vi "Get Codec.vi"(8 "error in (no error)":errorcluster, 10 "Codec In":string, 11 "Absolute Path":path) -> (0 "error out":errorcluster, 3 "Codec Out":string)   [LabVIEW 2020, in "G-Audio.lvlib"]
doc: "Determines supported audio codec name based on file extension or wired in codec string."
uses:
  G-Audio.lvlib
  <vilib>/Utility/error.llb/Error Cluster From Error Code.vi
  <vilib>/ErrorRing/Error Ring.xnode
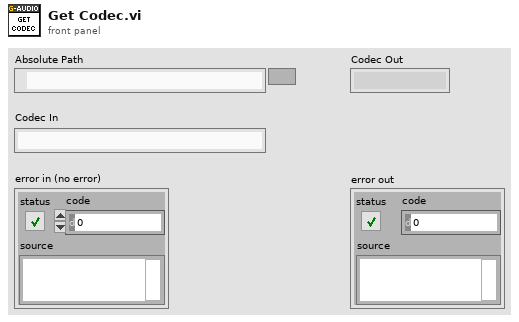
[diagram p1: front panel]
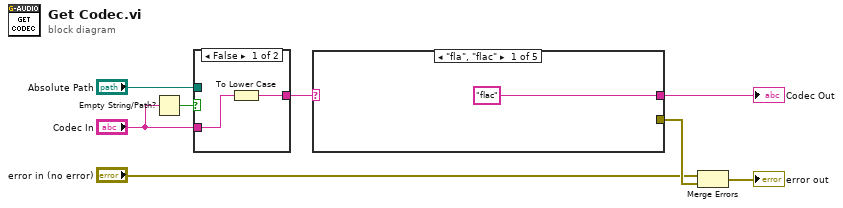
[diagram p0: block diagram]
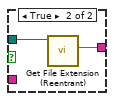
[diagram p2: hidden frame]
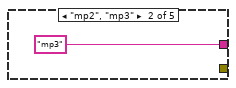
[diagram p3: hidden frame]
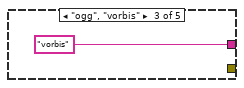
[diagram p4: hidden frame]
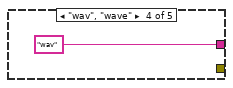
[diagram p5: hidden frame]
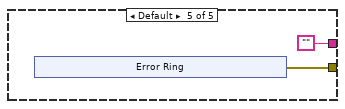
[diagram p6: hidden frame]
diagram:
  n1 = Empty String/Path?(string/path="Codec In") -> (empty?=w8:bool)
  n2 = case shown="False" w8 {
    tunnel: "Absolute Path" -> [_ w12]
    tunnel: [w9 w11] -> w6
    tunnel: "Codec In" -> [w10 _]
    frame False {
      n3 = To Lower Case(string=w10) -> (all lower case string=w9:string)
    }
    frame True {
      n4 = call "Get File Extension (Reentrant).vi"("file"=w12) -> ("lowercase file extension"=w11:string)  [unwired: 6 in, 4 out]
    }
  }
  n5 = case shown="\"fla\", \"flac\"" w6 {
    tunnel: ["flac" ("lowercase file extension") "mp3" ("lowercase file extension") "vorbis" ("lowercase file extension") "wav" ("lowercase file extension") "" ("lowercase file extension")] -> w4
    tunnel: [_ _ _ _ w17] -> w3
    frame "fla", "flac" {
    }
    frame "mp2", "mp3" {
    }
    frame "ogg", "vorbis" {
    }
    frame "wav", "wave" {
    }
    frame Default {
      n6 = xnode ("Error Ring")() -> ("error out"=w17:errorcluster)
    }
  }
  "Codec Out" <- w4
  n7 = Merge Errors("error in (no error)", w3) -> (→"error out":errorcluster)
